vi "CSGaussmeter.setRel.vi"(0 "i ref in":refnum<vi>, 7 "Rel":bool, 11 "error in (no error)":errorcluster) -> (4 "i ref out":refnum<vi>, 15 "error out":errorcluster)   [LabVIEW 2014, in "CSGaussmeter.lvlib"]
doc: "This VI sets the Relative ON or OFF. \n\nDas VI Rel wird zum Ein- bzw. Ausschalten der Relativ-Funktion verwendet. Mit der Funktion Relative können kleine Änderungen in großen Magnetfeldern leichter beobachtet werden. Ist die Funktion eingeschaltet, werden nur die Abweichungen von einem zuvor gewählten Bezugswert angezeigt."
uses:
  CSGaussmeter.lvlib
  CSCore/CSObj/CSObj.lvlib
  CSlibraries/UtilityLib/UtilityLib.lvlib
  CSinstr.lib/FH_55/FH 55.lvlib
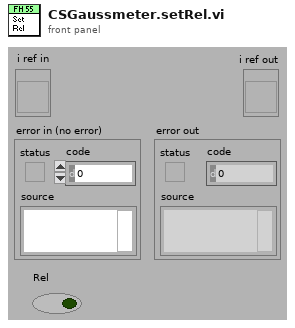
[diagram p1: front panel]
types:
  T1 = typedef "CSGaussmeter.lvlib/CSGaussmeter.i attribute.ctl" = cluster{"Name":string, "VISA Resource Name":refnum<visa-resource-name>, "actValues":cluster{" Limit":bool, "Unit ":T2, "Temp_Unit":T3, "Max":T4, " Filter":bool, " Peak":bool, " Auto_Range":bool, "Range":T5, " Rel":bool, " CTemp":bool, " CField":bool, "AC_DC ":bool, "Set_lower":cluster{"Numeric":dbl, "Cancel Button":bool, "Unit":T6}, "Set_upper":cluster{"Numeric":dbl, "Cancel Button":bool, "Unit":T6}, "Set_Rel":cluster{"Numeric":dbl, "Cancel Button":bool, "Unit":T6}, "Zero":bool, " Local":bool, "Reset":bool, " Init":bool}, "FH 55 Gauss-/Teslameter":T7, "MAX_Value":T8, "MIN_Value":T8, "Rel_Value":T8, "Array ":string[], "LIMU":dbl, " LIML":dbl, "Messwerte 2":string, "Messwerte ":cluster{"Numeric":i32, "OK Button":bool}, "serviceID":cluster{"Current ID":i32, "Unit ID":i32, "Temp ID":i32, "Name ID \n":i32, "Visa ID ":i32}, "setValues ":cluster{" Limit":bool, "Unit ":T2, "Temp_Unit":T3, "Max":T4, " Filter":bool, " Peak":bool, " Auto_Range":bool, "Range":T5, " Rel":bool, " CTemp":bool, " CField":bool, "AC_DC ":bool, "Set_lower":cluster{"Numeric":dbl, "Cancel Button":bool, "Unit":T6}, "Set_upper":cluster{"Numeric":dbl, "Cancel Button":bool, "Unit":T6}, "Set_Rel":cluster{"Numeric":dbl, "Cancel Button":bool, "Unit":T6}, "Zero":bool, " Local":bool, "Reset":bool, " Init":bool}}
  T2 = typedef "FH 55.lvlib/Unit.ctl" = enum16{"T", "G", "A/m"}
  T3 = typedef "FH 55.lvlib/Temp_Unit.ctl" = enum16{"Temp off", "Celsius", "Fahrenheit"}
  T4 = typedef "FH 55.lvlib/Max.ctl" = enum16{"MAX off", "Show MAX", "MAX/MIN"}
  T5 = typedef "FH 55.lvlib/Range.ctl" = enum16{"1", "2", "3", "4", "5", "6", "7"}
  T6 = typedef "FH 55.lvlib/Unit2.ctl" = enum16{"mT", "G", "kA/m"}
  T7 = typedef "FH 55.lvlib/Display.ctl" = cluster{"current value":string, "Limit":string, "Remote":string, "function ":string, "Cluster":cluster{"AC/DC":string, "Auto":string, "Filter":string, "Range":string, "Rel":string, "Peak":string}}
  T8 = typedef "FH 55.lvlib/Value_String.ctl" = cluster{"Numeric":dbl, "String":string}
  T9 = cluster{"VISA Resource Name":refnum<visa-resource-name>}
  T10 = typedef "FH 55.lvlib/VisaCluster.ctl" = cluster{"VISA Resource Name":refnum<visa-resource-name>}
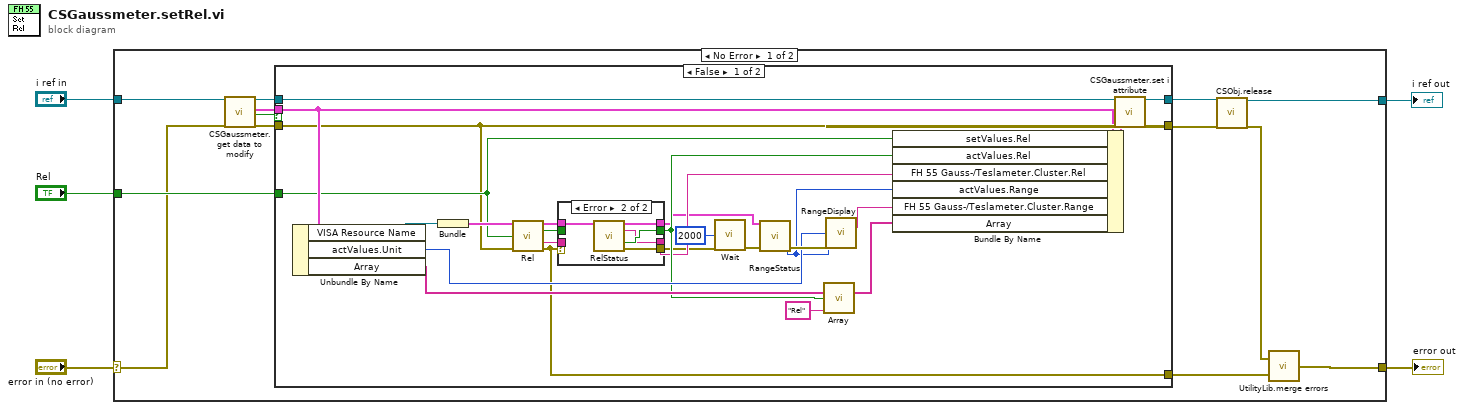
[diagram p0: block diagram]
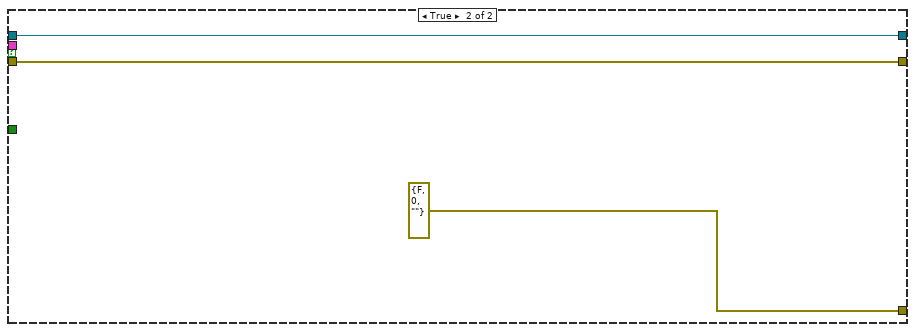
[diagram p3: hidden frame]
diagram:
  n1 = case shown="No Error" "error in (no error)" {
    selector: "error in (no error)" -> [w12 w57]
    tunnel: [w13 w57] -> w2
    tunnel: "i ref in" -> [w11 w58]
    tunnel: [w6 w58] -> w3
    tunnel: "Rel" -> [w15 _]
    frame No Error {
      n2 = call "CSGaussmeter.get data to modify.vi"("i ref in"=w11, "error in (no error)"=w12) -> ("i ref out"=w10:refnum<vi>, "i attribute"=w9:T1, "timed out"=w8:bool, "error out"=w7:errorcluster)  [unwired: 14 in]
      n3 = case shown="False" w8 {
        tunnel: w10 -> [w42 w55]
        tunnel: w7 -> [w36 w56]
        tunnel: w9 -> [w43 _]
        tunnel: [w35 w56] -> w16
        tunnel: [w40 w55] -> w18
        tunnel: w15 -> [w38 _]
        tunnel: [w23 errorcluster {"status"=FALSE, "code"=0, "source"=""} ("error out")] -> w14
        frame False {
          n4 = Unbundle By Name(w43) -> ("VISA Resource Name"=w44:refnum<visa-resource-name>, "actValues.Unit"=w32:T2, "Array"=w29:string[])
          n5 = Bundle("VISA Resource Name"=w44) -> (w39:T9)  [unwired: 1 in]
          n6 = call "Rel.vi"("VisaCluster"=w39, "Rel"=w38, "error in (no error)"=w36) -> ("VisaCluster"=w28:T10, "Boolean"=w27:bool, "Display"=w25:string, "error out"=w23:errorcluster)  [unwired: 8 in, 1 out]
          n7 = case shown="Error" w23 {
            selector: w23 -> [w45 _]
            tunnel: w28 -> [w48 w49]
            tunnel: [w48 w53] -> w22
            tunnel: w27 -> [w47 _]
            tunnel: [w47 w52] -> w26
            tunnel: [w46 w51] -> w24
            tunnel: w25 -> [w46 _]
            tunnel: [w45 w50] -> w21
            frame No Error {
            }
            frame Error {
              n8 = call "RelStatus.vi"("VisaCluster"=w49) -> ("VisaCluster"=w53:T10, "Display"=w51:string, "Rel"=w52:bool, "error out"=w50:errorcluster)  [unwired: 10 in, 1 out]
            }
          }
          n9 = call "Wait.vi"("milliseconds to wait"=u32 2000, "error in (no error)"=w21) -> ("error out"=w20:errorcluster)  [unwired: 13 in]
          n10 = call "RangeStatus.vi"("VisaCluster"=w22, "error in (no error)"=w20) -> ("Range"=w31:T5, "error out"=w33:errorcluster)  [unwired: 10 in, 2 out]
          n11 = call "Array.vi"("Array"=w29, "Boolean"=w26, "String"="Rel" ("element")) -> ("Array"=w34:string[])  [unwired: 12 in]
          n12 = call "RangeDisplay.vi"("Unit"=w32, "Range"=w31, "error in (no error)"=w33) -> ("Display"=w30:string)  [unwired: 10 in, 2 out]
          n13 = Bundle By Name(cluster=w43, "setValues.Rel"=w38, "actValues.Rel"=w26, "FH 55 Gauss-/Teslameter.Cluster.Rel"=w24, "actValues.Range"=w31, "FH 55 Gauss-/Teslameter.Cluster.Range"=w30, "Array"=w34) -> (w41:T1)
          n14 = call "CSGaussmeter.set i attribute.vi"("i ref in"=w42, "i attribute"=w41, "error in (no error)"=w36) -> ("i ref out"=w40:refnum<vi>, "error out"=w35:errorcluster)  [unwired: 15 in]
        }
        frame True {
        }
      }
      n15 = call "CSObj.release.vi"("i ref in"=w18, "error in (no error)"=w16) -> ("i ref out"=w6:refnum<vi>, "error out"=w17:errorcluster)  [unwired: 16 in]
      n16 = call "UtilityLib.merge errors.vi"("error2 (no error)"=w14, "error1 (no error)"=w17) -> ("error out"=w13:errorcluster)
    }
    frame Error {
    }
  }
  "i ref out" <- w3
  "error out" <- w2
